vi "BLValve_control.vi"(4 "FieldPoint IO Point 2":refnum<k21>, 6 "FieldPoint IO Point 3":refnum<k21>, 7 "OK Button 7":bool, 9 "FieldPoint IO Point":refnum<k21>, 10 "reference in":refnum<vi>, 11 "Boolean in":refnum<vi>) -> (0 "error out":errorcluster, 1 "BL Open":errorcluster caption="error out", 2 "BL Close":errorcluster caption="error out", 3 "Boolean 11":bool, 5 "Boolean 12":bool)   [LabVIEW 2014]
uses:
  <vilib>/FieldPoint/Polymorphic Read.llb/FP Read (Boolean -IO).vi
  <vilib>/FieldPoint/Polymorphic Write.llb/FP Write (Boolean -IO).vi
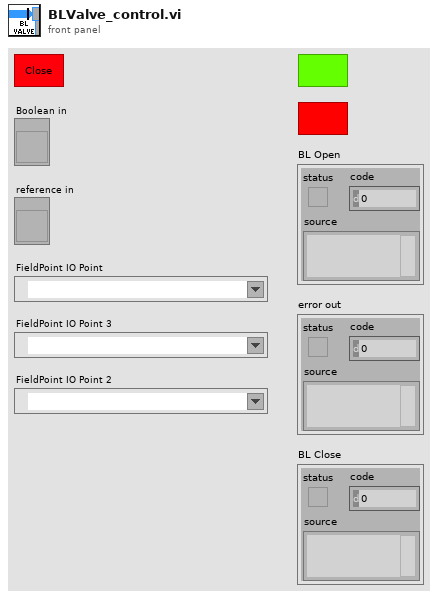
[diagram p1: front panel]
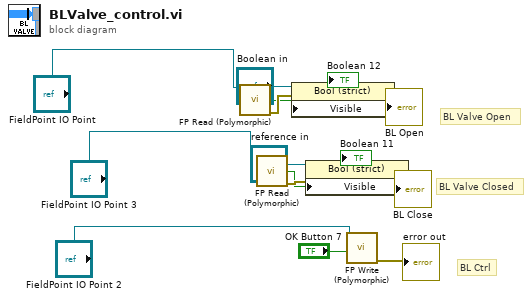
[diagram p0: block diagram]
diagram:
  # "BL Ctrl"
  # "BL Valve Closed"
  # "BL Valve Open"
  n1 = call-poly <vilib>:"FP Read (Polymorphic).vi"("FieldPoint IO Point In"="FieldPoint IO Point") -> ("value"=w6:bool, "error out"=w9:errorcluster)  [unwired: 11 in, 2 out]
  n2 = call-poly <vilib>:"FP Read (Polymorphic).vi"("FieldPoint IO Point In"="FieldPoint IO Point 3") -> ("value"=w8:bool, "error out"=w11:errorcluster)  [unwired: 11 in, 2 out]
  n3 = property on="Property Node" class="Bool (strict)"(reference="Boolean in", error in=w9, "Visible"=w6) -> (error out=→"BL Open":errorcluster)  [unwired: 1 out]
  n4 = property on="Property Node" class="Bool (strict)"(reference="reference in", error in=w11, "Visible"=w8) -> (error out=→"BL Close":errorcluster)  [unwired: 1 out]
  n5 = call-poly <vilib>:"FP Write (Polymorphic).vi"("FieldPoint IO Point In"="FieldPoint IO Point 2", "value"="OK Button 7") -> ("error out"=→"error out":errorcluster)  [unwired: 11 in, 2 out]
